vi "CSV Headings.vi"(9 "Heading 2":string, 11 "Heading 1":string) -> (2 "CSV Heading String":string)   [LabVIEW 2021]
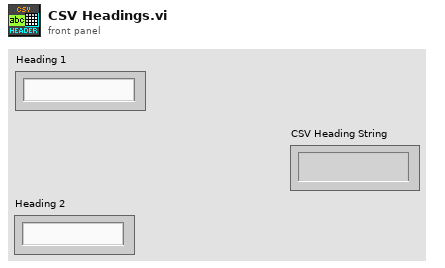
[diagram p1: front panel]
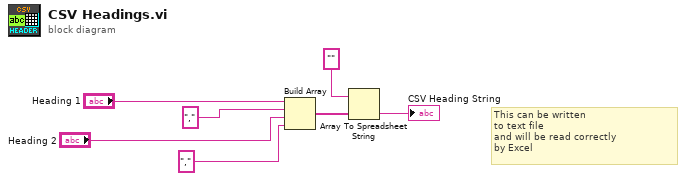
[diagram p0: block diagram]
diagram:
  # "This can be written\nto text file\nand will be read correctly\nby Excel"
  n1 = Build Array("Heading 1", "," ("element"), "Heading 2", "," ("element")) -> (w5:string[])
  n2 = Array To Spreadsheet String(array=w5, 3:"" ("format string")) -> (spreadsheet string=→"CSV Heading String":string)  [unwired: 1 in]
